vi "Rotate Image.vi"(8 "error in (no error)":errorcluster, 10 "Degrees":dbl, 11 "Image":T1) -> (0 "error out":errorcluster, 3 "Rotated Image":T1)   [LabVIEW 2020, in "G-Image.lvlib"]
doc: "Rotate the image by the specified number of degrees."
uses:
  G-Image.lvlib
  <vilib>/picture/picture.llb/imagedata.ctl
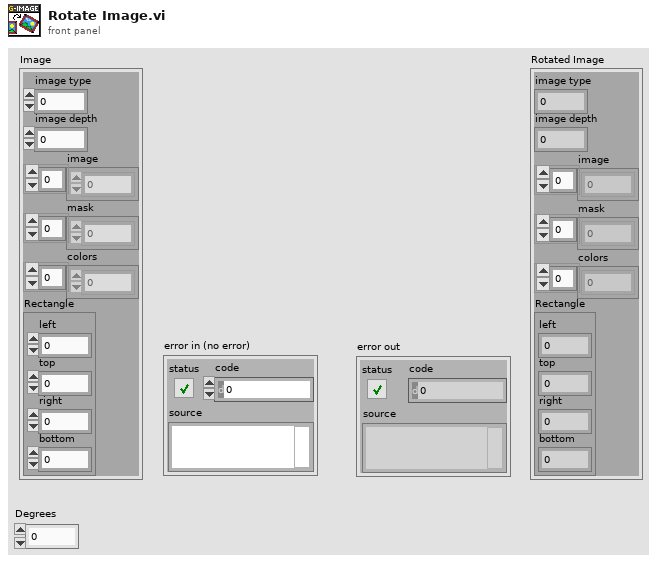
[diagram p1: front panel]
types:
  T1 = typedef "imagedata.ctl" = cluster{"image type":i32, "image depth":i32, "image":u8[], "mask":u8[], "colors":u32[], "Rectangle":cluster{"left":i16, "top":i16, "right":i16, "bottom":i16}}
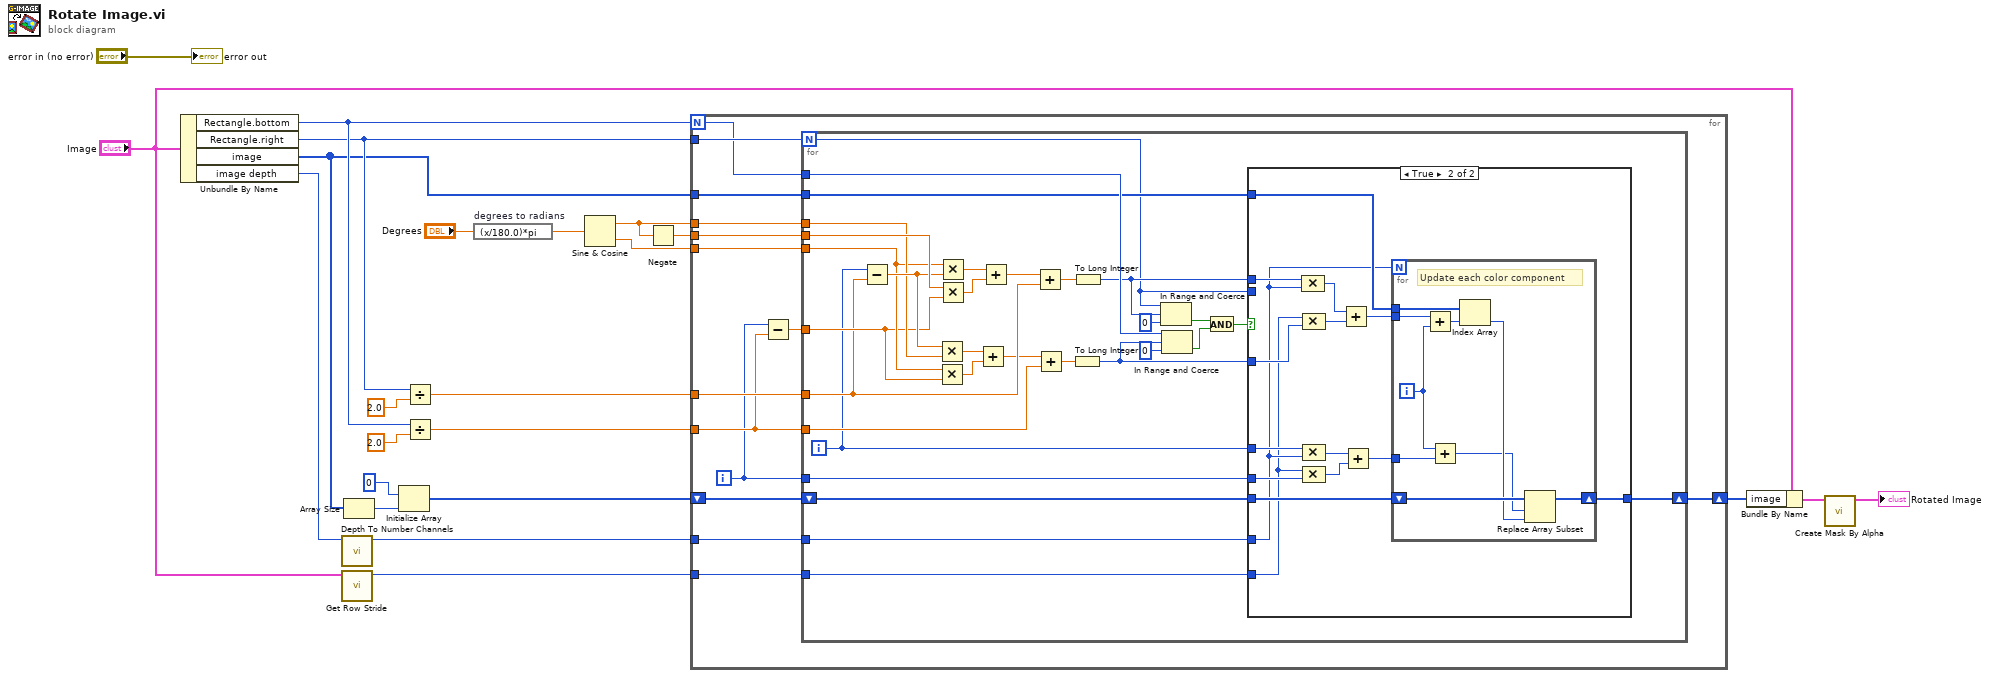
[diagram p0: block diagram]
diagram:
  n1 = Unbundle By Name("Image") -> ("Rectangle.bottom"=w23:i16, "Rectangle.right"=w22:i16, "image"=w19:u8[], "image depth"=w4:i32)
  n2 = call "Depth To Number Channels.vi"("Depth"=w4) -> ("Channels"=w3:i32)  [unwired: 10 in]
  n3 = call "Get Row Stride.vi"("Image"="Image") -> ("Row Stride"=w1:i32)  [unwired: 9 in, 1 out]
  n4 = Array Size(array=w19) -> (size(s)=w21:i32)
  n5 = Initialize Array(u8 0, w21) -> (w18:u8[])
  n6 = Divide(x=w22, y=2.0) -> (x/y=w15:dbl)
  n7 = Divide(x=w23, y=2.0) -> (x/y=w14:dbl)
  n8 = expression code="(x/180.0)*pi" "degrees to radians"("Degrees") -> (w13:dbl)
  n9 = Sine & Cosine(0:w13) -> (1:w10:dbl, 2:w12:dbl)
  n10 = Negate(x=w10) -> (-x=w11:dbl)
  n11 = for {
    N: w23 -> [w29]
    tunnel: w22 -> [w37]
    tunnel: w19 -> [w36]
    tunnel: w15 -> [w35]
    tunnel: w14 -> [w34]
    tunnel: w12 -> [w32]
    tunnel: w11 -> [w31]
    tunnel: w10 -> [w30]
    shift-right: [w26] -> w9
    shift-left: w18 -> [w27]
    tunnel: w3 -> [w25]
    tunnel: w1 -> [w24]
    i -> [w28]
    n12 = Subtract(x=w28, y=w34) -> (x-y=w33:dbl)
    n13 = for {
      N: w37 -> [w47]
      tunnel: w36 -> [w50]
      tunnel: w35 -> [w58]
      tunnel: w34 -> [w56]
      tunnel: w33 -> [w62]
      tunnel: w32 -> [w63]
      tunnel: w31 -> [w68]
      tunnel: w30 -> [w64]
      tunnel: w29 -> [w53]
      tunnel: w28 -> [w45]
      shift-right: [w43] -> w26
      shift-left: w27 -> [w44]
      tunnel: w25 -> [w40]
      tunnel: w24 -> [w38]
      i -> [w46]
      n14 = Subtract(x=w46, y=w58) -> (x-y=w65:dbl)
      n15 = Multiply(x=w65, y=w64) -> (x*y=w61:dbl)
      n16 = Multiply(x=w63, y=w62) -> (x*y=w60:dbl)
      n17 = Multiply(x=w63, y=w65) -> (x*y=w67:dbl)
      n18 = Multiply(x=w68, y=w62) -> (x*y=w66:dbl)
      n19 = Add(x=w61, y=w60) -> (x+y=w57:dbl)
      n20 = Add(x=w67, y=w66) -> (x+y=w59:dbl)
      n21 = Add(x=w59, y=w58) -> (x+y=w55:dbl)
      n22 = Add(x=w57, y=w56) -> (x+y=w54:dbl)
      n23 = To Long Integer(number=w54) -> (32bit integer=w48:i32)
      n24 = To Long Integer(number=w55) -> (32bit integer=w49:i32)
      n25 = In Range and Coerce(upper limit=w47, x=w49, lower limit=0) -> (In Range?=w52:bool)  [unwired: 1 out]
      n26 = In Range and Coerce(upper limit=w53, x=w48, lower limit=0) -> (In Range?=w51:bool)  [unwired: 1 out]
      n27 = And(x=w52, y=w51) -> (x .and. y?=w39:bool)
      n28 = case shown="True" w39 {
        tunnel: w50 -> [_ w84]
        tunnel: w49 -> [_ w81]
        tunnel: w48 -> [_ w83]
        tunnel: w47 -> [_ _]
        tunnel: w46 -> [_ w77]
        tunnel: w45 -> [_ w79]
        tunnel: w44 -> [w69 w76]
        tunnel: [w69 w75] -> w43
        tunnel: w40 -> [_ w71]
        tunnel: w38 -> [_ w70]
        frame False {
        }
        frame True {
          n29 = Compound Arithmetic op=MULTIPLY(w81, w71) -> (w72:i32)
          n30 = Compound Arithmetic op=MULTIPLY(w70, w83) -> (w82:i32)
          n31 = Compound Arithmetic op=MULTIPLY(w77, w71) -> (w73:i32)
          n32 = Compound Arithmetic op=MULTIPLY(w70, w79) -> (w78:i32)
          n33 = Add(x=w72, y=w82) -> (x+y=w80:i32)
          n34 = Add(x=w73, y=w78) -> (x+y=w74:i32)
          n35 = for {
            N: w71 -> [_]
            tunnel: w84 -> [w93]
            tunnel: w80 -> [w87]
            tunnel: w74 -> [w89]
            shift-right: [w91] -> w75
            shift-left: w76 -> [w92]
            i -> [w86]
            # "Update each color component"
            n36 = Add(x=w87, y=w86) -> (x+y=w85:i32)
            n37 = Add(x=w86, y=w89) -> (x+y=w88:i32)
            n38 = Index Array(array=w93, index=w85) -> (element=w90:u8)
            n39 = Replace Array Subset(array=w92, new element=w90, index=w88) -> (w91:u8[])
          }
        }
      }
    }
  }
  n40 = Bundle By Name(cluster="Image", "image"=w9) -> (w7:T1)
  n41 = call <vilib>:"Create Mask By Alpha.vi"("image data"=w7) -> ("masked image data"=→"Rotated Image":T1)  [unwired: 10 in]
  "error out" <- "error in (no error)"
